vi "GPIB Write OnlyOF.vi"(4 "Command String":string, 5 "GPIB Card":i16 min=0 max=3, 6 "GPIB Address":i16=15 max=30 step=1) -> (2 "Write Status":string)   [LabVIEW 2023]
doc: "GPIB Fetch sends the Command String to the Addressed GPIB device, then reads the data back placing the results in Characters Read. Status strings are available for both read & write operations."
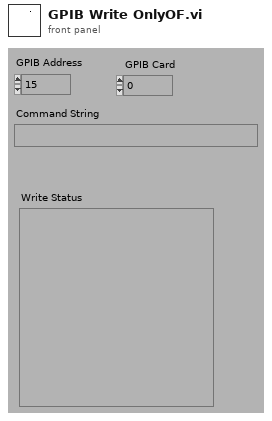
[diagram p1: front panel]
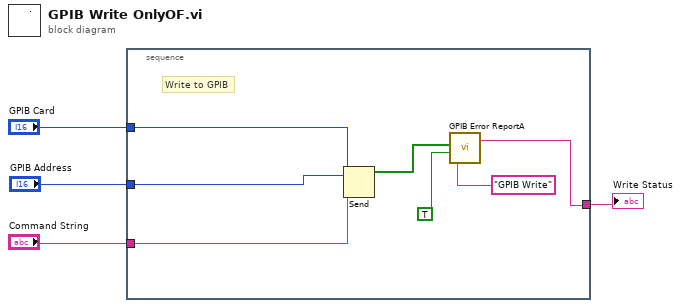
[diagram p0: block diagram]
diagram:
  n1 = stacked-sequence {
    tunnel: "Command String" -> [w8]
    tunnel: [w5] -> w4
    tunnel: "GPIB Card" -> [w7]
    tunnel: "GPIB Address" -> [w6]
    frame #0 {
      # "Write to GPIB"
      n2 = Send(0:w7, 2:w6, 5:w8) -> (6:w11:bool[])  [unwired: 2 in, 2 out]
      n3 = call "GPIB Error ReportA.vi"("Function"="GPIB Write", "Dialog?(F)"=TRUE, "Status"=w11) -> ("Status String"=w5:string)  [unwired: 1 in, 1 out]
    }
  }
  "Write Status" <- w4
